vi "Recover Files.vi"(6 "Error Message in":string, 8 "Error In":errorcluster, 9 "Full App Name":string="PC Interface.exe", 10 "Temp path Array":path[](array[path]), 11 "Server Files Cluster":T1) -> (0 "Error Out":errorcluster, 3 "Files Recovered":bool, 4 "Error Message out":string)   [LabVIEW 2019]
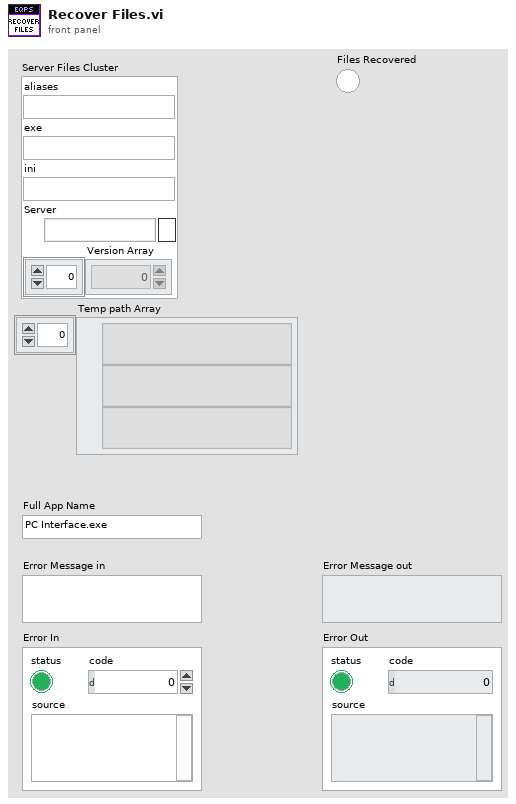
[diagram p1: front panel]
types:
  T1 = cluster{"aliases":string, "exe":string, "ini":string, "Server":path, "Version Array":i32[]}
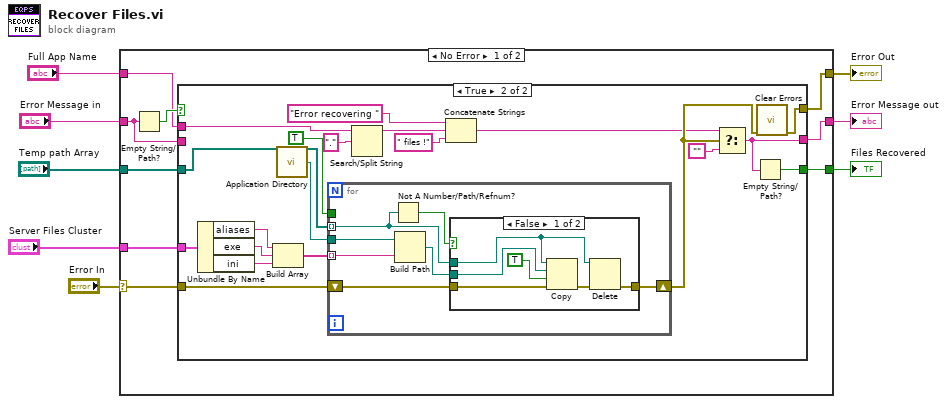
[diagram p0: block diagram]
diagram:
  n1 = case shown="No Error" "Error In" {
    selector: "Error In" -> [w13 w55]
    tunnel: [w14 w55] -> w7
    tunnel: [w16 w54] -> w6
    tunnel: "Error Message in" -> [w15 w54]
    tunnel: "Server Files Cluster" -> [w12 _]
    tunnel: [w11 _] -> w3
    tunnel: "Temp path Array" -> [w10 _]
    tunnel: "Full App Name" -> [w9 _]
    frame No Error {
      n2 = Empty String/Path?(string/path=w15) -> (empty?=w17:bool)
      n3 = case shown="True" w17 {
        tunnel: [w19 w29] -> w16
        tunnel: w15 -> [w19 _]
        tunnel: [w18 w31] -> w14
        tunnel: w13 -> [w18 w28]
        tunnel: w12 -> [_ w38]
        tunnel: [_ w30] -> w11
        tunnel: w10 -> [_ w27]
        tunnel: w9 -> [_ w24]
        frame False {
        }
        frame True {
          n4 = Unbundle By Name(w38) -> ("aliases"=w35:string, "exe"=w37:string, "ini"=w36:string)
          n5 = Build Array(w35, w37, w36) -> (w34:string[])
          n6 = call <vilib>:"Application Directory.vi"() -> ("Application Directory"=w39:path)
          n7 = for {
            tunnel: w39 -> [w46]
            tunnel: w34 -> [w45] mode=indexing
            shift-right: [w40] -> w26
            shift-left: w28 -> [w44]
            tunnel: TRUE ("overwrite (F)") -> [_]
            tunnel: w27 -> [w42] mode=indexing
            n8 = Not A Number/Path/Refnum?(number/path/refnum=w42) -> (NaN/Path/Refnum?=w43:bool)
            n9 = Build Path(base path=w46, name or relative path=w45) -> (appended path=w41:path)
            n10 = case shown="False" w43 {
              tunnel: w44 -> [w52 w53]
              tunnel: w42 -> [w47 _]
              tunnel: w41 -> [w51 _]
              tunnel: [w48 w53] -> w40
              frame False {
                n11 = Copy(8:w52, 9:TRUE ("overwrite (F)"), 10:w51, 11:w47) -> (0:w49:errorcluster)  [unwired: 1 in, 2 out]
                n12 = Delete(path (use dialog)=w47, error in=w49) -> (error out=w48:errorcluster)  [unwired: 3 in, 2 out]
              }
              frame True {
              }
            }
          }
          n13 = Search/Split String(string=w24, search string/char (-)=".") -> (substring before match=w20:string)  [unwired: 1 in, 2 out]
          n14 = Concatenate Strings("Error recovering ", w20, " files !") -> (w23:string)
          n15 = Select(t=w23, s=w26, f="") -> (s? t:f=w29:string)
          n16 = Empty String/Path?(string/path=w29) -> (empty?=w30:bool)
          n17 = call <vilib>:"Clear Errors.vi"("error in (no error)"=w26) -> ("error out"=w31:errorcluster)  [unwired: 5 in, 1 out]
        }
      }
    }
    frame Error {
    }
  }
  "Error Out" <- w7
  "Error Message out" <- w6
  "Files Recovered" <- w3
